vi "Create xls File.vi"(4 "error in":errorcluster, 5 "Folder":T1) -> (0 "error out":errorcluster, 1 "Valid File":bool, 2 "path":path, 3 "refnum":refnum<file>)   [LabVIEW 2015]
uses:
  Process Controller 3.0/Calibration and Function folders.ctl
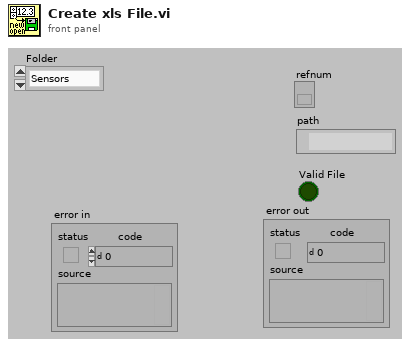
[diagram p1: front panel]
types:
  T1 = typedef "Calibration and Function folders.ctl" = enum16{"Sensors", "Functions", "Config File", "PublicAppFolder", "New ini File", "Set Config File", "Delete ini File"}
  T2 = enum16{"open", "open or create", "create or replace", "create", "open (read only)"}
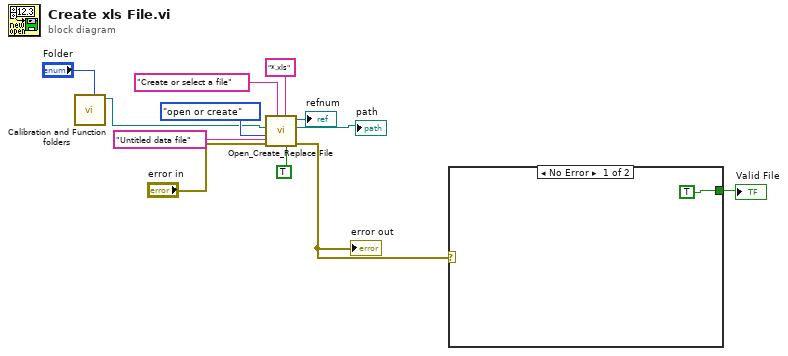
[diagram p0: block diagram]
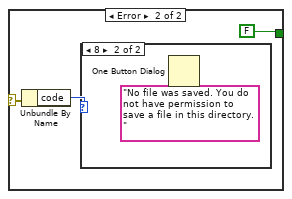
[diagram p2: hidden frame]
diagram:
  n1 = call "Calibration and Function folders.vi"("Folder"="Folder") -> ("Selected Folder"=w2:path)  [unwired: 9 in, 1 out]
  n2 = call <vilib>:"Open_Create_Replace File.vi"("advisory dialog? (display:T)"=TRUE, "pattern"="*.xls", "default name"="Untitled data file", "prompt"="Create or select a file", "error in (no error)"="error in", "function (open:0)"=T2."open or create", "start path  (Not A Path)"=w2) -> ("error out"=w6:errorcluster, "new file path"=→"path":path, "refnum"=→"refnum":refnum<file>)  [unwired: 1 in, 1 out]
  "error out" <- w6
  n3 = case shown="No Error" w6 {
    selector: w6 -> [_ w16]
    tunnel: [TRUE ("Valid File") FALSE ("Valid File")] -> w3
    frame No Error {
    }
    frame Error {
      n4 = Unbundle By Name(w16) -> ("code"=w15:i32)
      n5 = case shown="8" w15 {
        frame 0, Default {
        }
        frame 8 {
          n6 = One Button Dialog(message="No file was saved. You do not have permission to save a file in this directory.") -> ()  [unwired: 1 in, 1 out]
        }
      }
    }
  }
  "Valid File" <- w3
